vi "subPanelVertical.vi"() -> ()   [LabVIEW 2023, in "GUI.lvlib"]
uses:
  GUI.lvlib
panel:
  in  "Stop event":refnum<user-event>
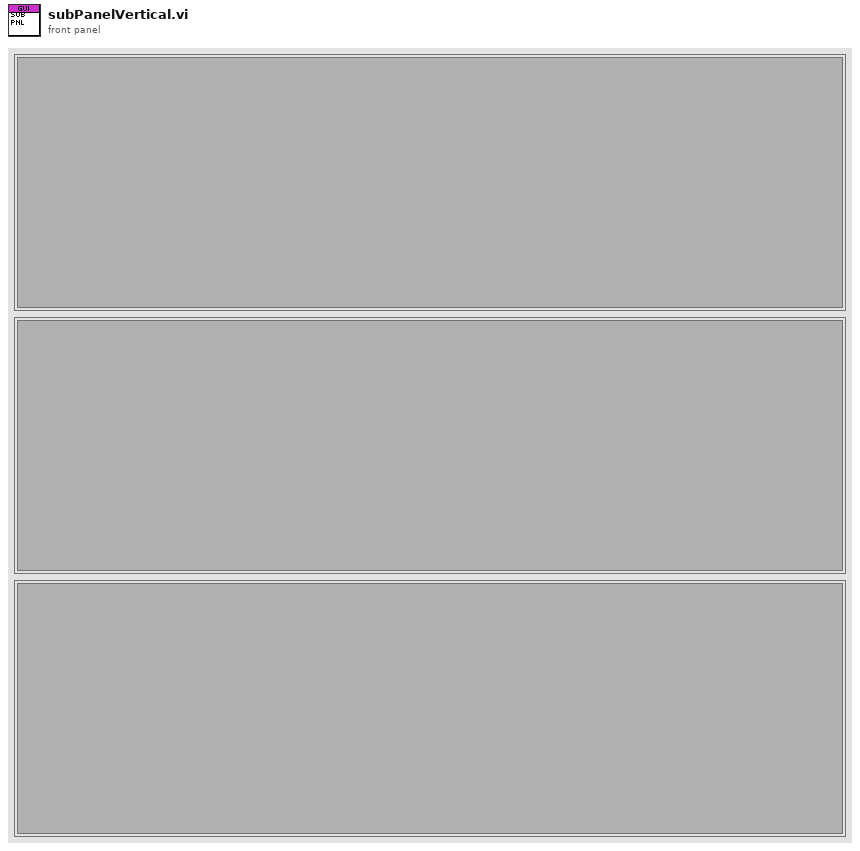
[diagram p1: front panel]
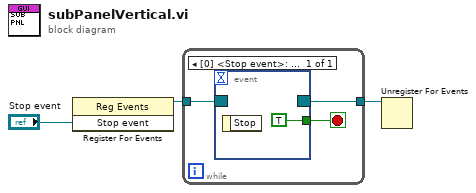
[diagram p0: block diagram]
diagram:
  n1 = register-events("Stop event") -> (reference out=w3:refnum<event-registration>)  [unwired: 2 in, 1 out]
  n2 = while {
    tunnel: w3 -> [w6]
    tunnel: [w5] -> w2
    stop <- w4 stop-if-true
    n3 = event shown="[0] <Stop event>: User Event" {
      selector: w6 -> [_]
      dyn-events: [_] -> w5
      timeout: _ -> [_]
      tunnel: [TRUE] -> w4
      event User Event {
        n4 = event-data() -> ()  [unwired: 2 out]
      }
    }
  }
  n5 = Unregister For Events(event registration refnum=w2) -> ()  [unwired: 1 in, 1 out]
